vi "DASI_MS2000.vi"() -> (2 "error out":errorcluster)   [LabVIEW 2011]
panel:
  out "has stopped":bool
  out "position":dbl[](array[numeric])
  out "Value":string="12.3"
  out "command":string="stage.x.set"
  # "asi.port=com3\nas usual scale is meter!"
  # "noch nicht getestet\nnoch nicht stage.x.speed.set"
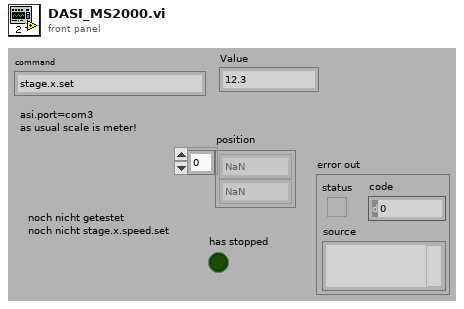
[diagram p1: front panel]
types:
  T1 = enum16{"None/#Datasets", "Clear", "TagValueOf#", "AddValues", "ReadValue", "ChangeValue", "Get all"}
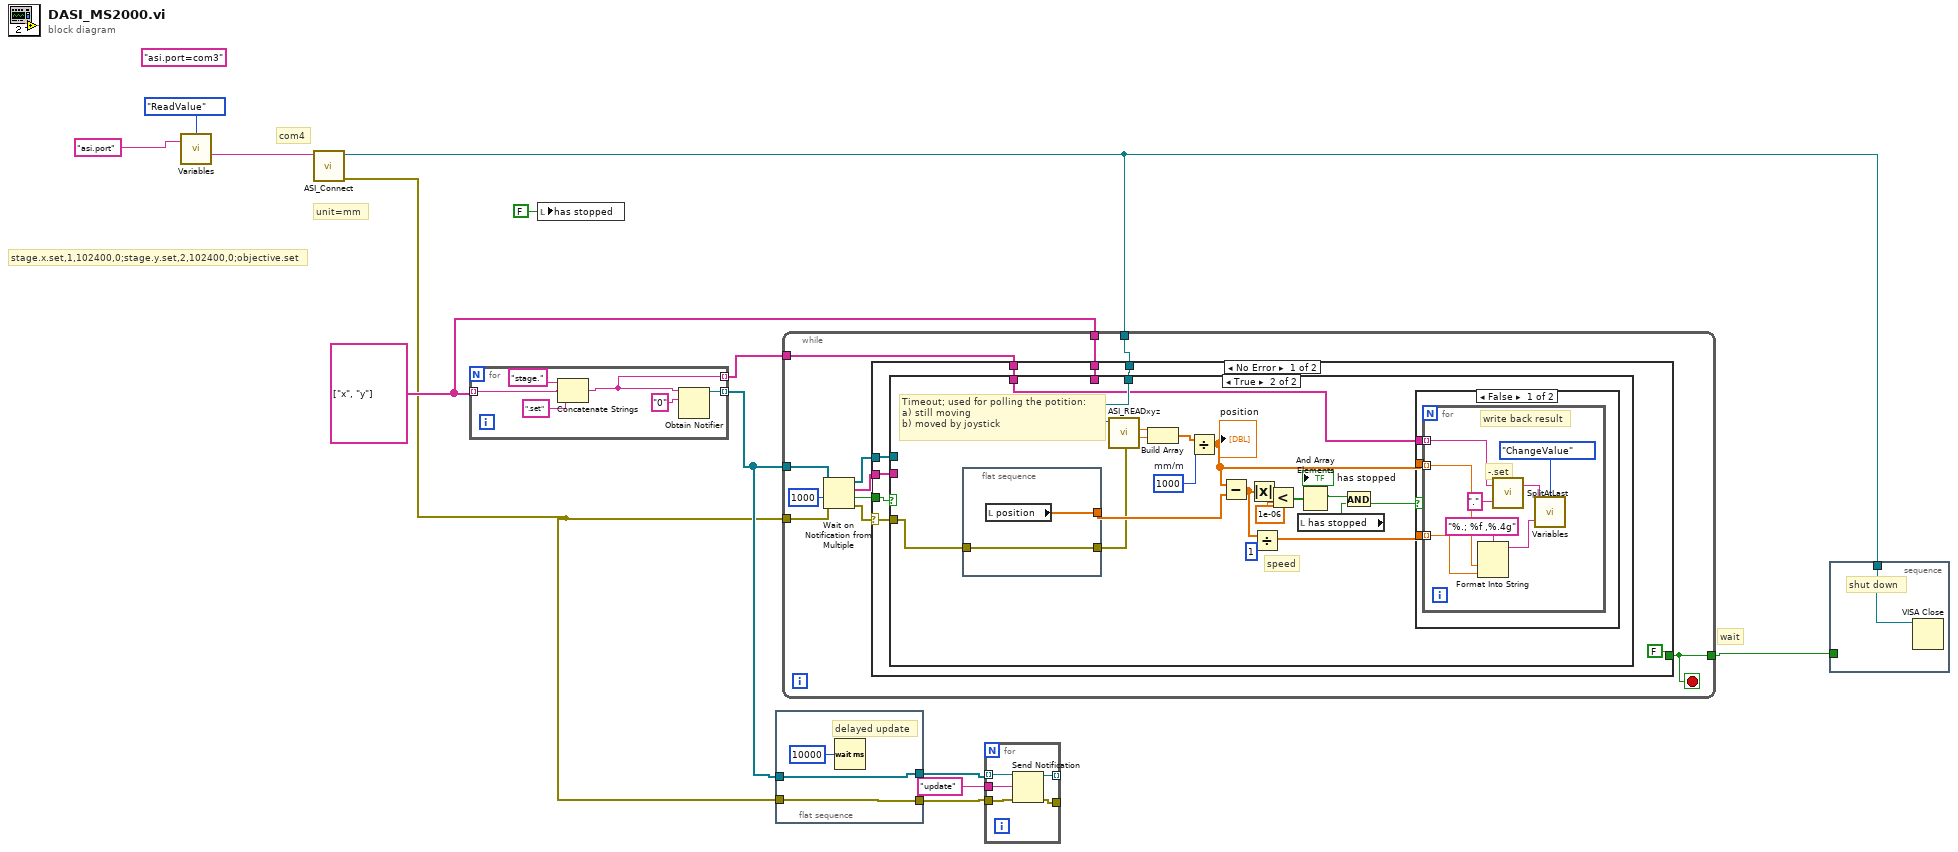
[diagram p0: block diagram]
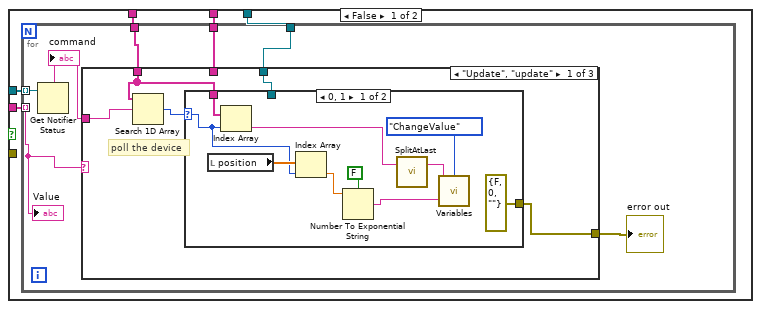
[diagram p2: hidden frame]
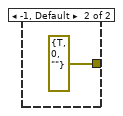
[diagram p3: hidden frame]
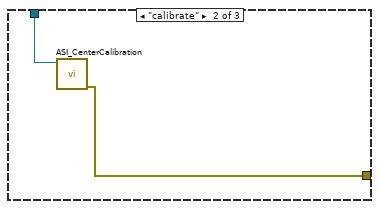
[diagram p4: hidden frame]
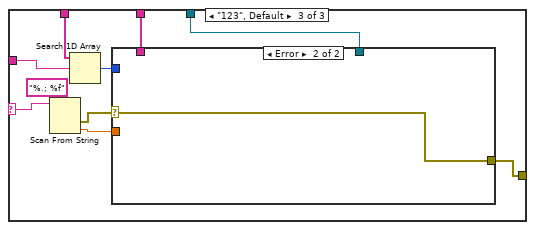
[diagram p5: hidden frame]
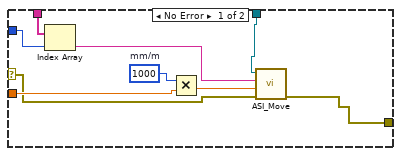
[diagram p6: hidden frame]
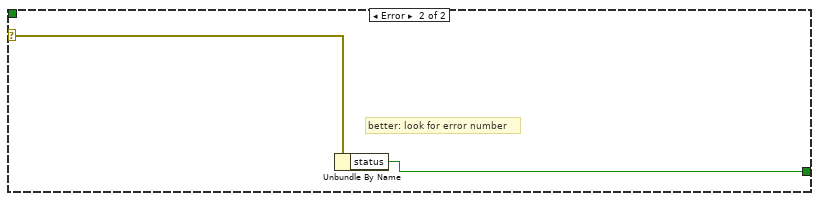
[diagram p8: hidden frame]
diagram:
  w3 = string[] ["x", "y"]
  (unwired) "asi.port=com3" ("Config-String")
  # "com4"
  # "stage.x.set,1,102400,0;stage.y.set,2,102400,0;objective.set"
  # "unit=mm"
  # "wait"
  n1 = call "Variables.vi"("Tag in"="asi.port", "Command"=T1."ReadValue") -> ("value out"=w6:string)  [unwired: 1 in, 2 out]
  n2 = call "ASI_Connect.vi"("VISA resource name"=w6) -> ("error out"=w2:errorcluster, "VISA resource name out"=w5:refnum<visa-resource-name>)  [unwired: 9 in]
  n3 = for {
    tunnel: w3 -> [w15] mode=indexing
    tunnel: [w18] -> w9 mode=indexing
    tunnel: [w14] -> w4 mode=indexing
    n4 = Concatenate Strings("stage." ("string"), w15, ".set" ("string")) -> (w14:string)
    n5 = Obtain Notifier(name (unnamed)=w14, notification data type="0") -> (notifier out=w18:refnum<notifier>)  [unwired: 2 in, 2 out]
  }
  n6 = local write "has stopped"(FALSE ("has stopped")) -> ()
  n7 = flat-sequence {
    tunnel: w9 -> [w21]
    tunnel: [w21] -> w8
    tunnel: w2 -> [w20]
    tunnel: [w20] -> w7
    frame #0 {
      # "delayed update"
      n8 = Wait (ms)(milliseconds to wait=u32 10000 ("Zu wartende ms")) -> ()  [unwired: 1 out]
    }
  }
  n9 = while {
    tunnel: w9 -> [w33]
    tunnel: w2 -> [w29]
    tunnel: [w28] -> w13
    tunnel: w5 -> [w27]
    tunnel: w4 -> [w26]
    tunnel: w3 -> [w25]
    stop <- w28 stop-if-true
    n10 = Wait on Notification from Multiple(0:w33, 2:1000 ("timeout in ms (-1)"), 3:w29) -> (8:w31:refnum<notifier>[], 9:w30:string[], 10:w24:bool, 11:w32:errorcluster)  [unwired: 1 out]
    n11 = case shown="No Error" w32 {
      selector: w32 -> [w34 w125]
      tunnel: w31 -> [w41 _]
      tunnel: w30 -> [w40 _]
      tunnel: [FALSE ("status") w124] -> w28
      tunnel: w27 -> [w38 _]
      tunnel: w26 -> [w37 _]
      tunnel: w25 -> [w36 _]
      tunnel: w24 -> [w35 _]
      frame No Error {
        n12 = case shown="True" w35 {
          tunnel: w41 -> [w46 _]
          tunnel: w40 -> [w45 _]
          tunnel: w38 -> [w44 w110]
          tunnel: w37 -> [w43 w104]
          tunnel: w36 -> [w42 _]
          tunnel: w34 -> [_ w100]
          frame False {
            n13 = for {
              tunnel: w46 -> [w53] mode=indexing
              tunnel: w45 -> [w50] mode=indexing
              tunnel: w44 -> [w49]
              tunnel: w43 -> [w48]
              tunnel: w42 -> [w47]
              n14 = Get Notifier Status(notifier=w53) -> (notifier name=w52:string)  [unwired: 1 in, 4 out]
              "command" <- w52
              n15 = case shown="\"Update\", \"update\"" w50 {
                selector: w50 -> [_ _ w76]
                tunnel: w52 -> [w58 _ w81]
                tunnel: [w55 w70 w80] -> w51
                tunnel: w49 -> [w56 w71 w78]
                tunnel: w48 -> [w54 _ w79]
                tunnel: w47 -> [_ _ w77]
                frame "Update", "update" {
                  # "poll the device"
                  n16 = Search 1D Array(1D array=w54, element=w58) -> (index of element=w57:i32)  [unwired: 1 out]
                  n17 = case shown="0, 1" w57 {
                    selector: w57 -> [w66 _]
                    tunnel: [errorcluster {"status"=FALSE, "code"=0, "source"=""} ("error in (no error)") errorcluster {"status"=TRUE, "code"=0, "source"=""} ("error in (no error)")] -> w55
                    tunnel: w56 -> [_ _]
                    tunnel: w54 -> [w68 _]
                    frame 0, 1 {
                      n18 = local read "position"() -> (w67:dbl[])
                      n19 = Index Array(array=w68, index=w66) -> (element=w63:string)
                      n20 = Index Array(array=w67, index=w66) -> (element=w62:dbl)
                      n21 = Number To Exponential String(number=w62, 1:FALSE ("use system decimal point (T)")) -> (E-format string=w59:string)  [unwired: 2 in]
                      n22 = call "SplitAtLast.vi"("In-String"=w63) -> ("Front (default)"=w64:string)  [unwired: 1 in, 1 out]
                      n23 = call "Variables.vi"("value"=w59, "Tag in"=w64, "Command"=T1."ChangeValue") -> ()  [unwired: 3 out]
                    }
                    frame -1, Default {
                    }
                  }
                }
                frame "calibrate" {
                  n24 = call "ASI_CenterCalibration.vi"("VISA resource name"=w71) -> ("error out"=w70:errorcluster)  [unwired: 7 in, 3 out]
                }
                frame "123", Default {
                  n25 = Scan From String(format string="%.; %f", input string=w76) -> (error out=w72:errorcluster, output 1=w75:dbl)  [unwired: 3 in, 2 out]
                  n26 = Search 1D Array(1D array=w79, element=w81) -> (index of element=w73:i32)  [unwired: 1 out]
                  n27 = case shown="Error" w72 {
                    selector: w72 -> [w82 w91]
                    tunnel: [w88 w91] -> w80
                    tunnel: w75 -> [w90 _]
                    tunnel: w78 -> [w89 _]
                    tunnel: w77 -> [w85 _]
                    tunnel: w73 -> [w83 _]
                    frame No Error {
                      w87 = 1000  # mm/m
                      n28 = Index Array(array=w85, index=w83) -> (element=w84:string)
                      n29 = Multiply(x=w87, y=w90) -> (x*y=w86:dbl)
                      n30 = call "ASI_Move.vi"("error in (no error)"=w82, "Position [mm]"=w86, "Axis"=w84, "VISA resource name"=w89) -> ("error out"=w88:errorcluster)  [unwired: 6 in, 1 out]
                    }
                    frame Error {
                    }
                  }
                }
              }
              "error out" <- w51
              "Value" <- w50
            }
          }
          frame True {
            w106 = 1000  # mm/m
            # "speed"
            # "Timeout; used for polling the potition:\na) still moving\nb) moved by joystick"
            n31 = flat-sequence {
              tunnel: [w123] -> w105
              tunnel: w100 -> [w122]
              tunnel: [w122] -> w99
              frame #0 {
                n32 = local read "position"() -> (w123:dbl[])
              }
            }
            n33 = call "ASI_READxyz.vi"("error in (no error)"=w99, "VISA resource name"=w110) -> ("y [mm]"=w108:dbl, "x [mm]"=w109:dbl)  [unwired: 5 in, 3 out]
            n34 = Build Array(w109, w108) -> (w107:dbl[])
            n35 = Divide(x=w107, y=w106) -> (x/y=w103:dbl[])
            "position" <- w103
            n36 = Subtract(x=w103, y=w105) -> (x-y=w98:dbl[])
            n37 = Absolute Value(x=w98) -> (abs(x)=w92:dbl[])
            n38 = Divide(x=w98, y=1) -> (x/y=w102:dbl[])
            n39 = Less?(x=w92, y=1e-06) -> (x < y?=w96:bool[])
            n40 = local read "has stopped"() -> (w93:bool)
            n41 = And Array Elements(Boolean array=w96) -> (logical AND=w94:bool)
            "has stopped" <- w94
            n42 = And(x=w94, y=w93) -> (x .and. y?=w95:bool)
            n43 = case shown="False" w95 {
              tunnel: w104 -> [w113 _]
              tunnel: w103 -> [w112 _]
              tunnel: w102 -> [w111 _]
              frame False {
                n44 = for {
                  tunnel: w113 -> [w118] mode=indexing
                  tunnel: w112 -> [w117] mode=indexing
                  tunnel: w111 -> [w116] mode=indexing
                  # "write back result"
                  # "-.set"
                  n45 = Format Into String(format string="%.; %f ,%.4g", w117, w116) -> (resulting string=w114:string)  [unwired: 2 in, 1 out]
                  n46 = call "SplitAtLast.vi"("search char"=".", "In-String"=w118) -> ("Front (default)"=w120:string)  [unwired: 1 out]
                  n47 = call "Variables.vi"("value"=w114, "Tag in"=w120, "Command"=T1."ChangeValue") -> ()  [unwired: 3 out]
                }
              }
              frame True {
              }
            }
          }
        }
      }
      frame Error {
        # "better: look for error number"
        n48 = Unbundle By Name(w125) -> ("status"=w124:bool)
      }
    }
  }
  n49 = for {
    tunnel: w8 -> [w130] mode=indexing
    tunnel: w7 -> [w129]
    tunnel: [w128] -> _
    tunnel: [w127] -> _ mode=indexing
    tunnel: "update" -> [w126]
    n50 = Send Notification(notification=w126, notifier=w130, error in (no error)=w129) -> (notifier out=w127:refnum<notifier>, error out=w128:errorcluster)
  }
  n51 = stacked-sequence {
    tunnel: w13 -> [_]
    tunnel: w5 -> [w131]
    frame #0 {
      # "shut down"
      n52 = VISA Close(VISA resource name=w131) -> ()  [unwired: 1 in, 1 out]
    }
  }
